vi "Get Array Value at Index - String.vi"(0 "JSON Tree In (JSON Array)":variant, 5 "Index":i32, 9 "Default Value if JSON Null":string, 11 "error in (no error)":errorcluster) -> (4 "JSON Tree Out Passthrough":variant, 6 "String Value":string, 10 "is JSON Null?":bool, 15 "error out":errorcluster)   [LabVIEW 2015, in "i3-json.lvlib"]
doc: "Use this template to build a VI to use as a subVI."
uses:
  i3-json.lvlib
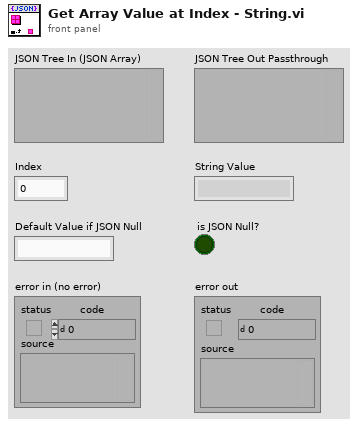
[diagram p1: front panel]
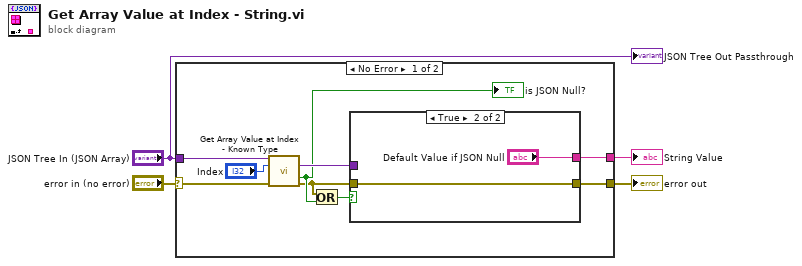
[diagram p0: block diagram]
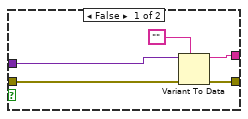
[diagram p2: hidden frame]
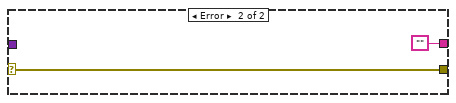
[diagram p3: hidden frame]
diagram:
  n1 = case shown="No Error" "error in (no error)" {
    selector: "error in (no error)" -> [w11 w22]
    tunnel: [w9 w22] -> w3
    tunnel: "JSON Tree In (JSON Array)" -> [w13 _]
    tunnel: [w6 ""] -> w2
    frame No Error {
      n2 = call "Get Array Value at Index - Known Type.vi"("JSON Tree In (JSON Array)"=w13, "Index"="Index", "error in (no error)"=w11) -> ("Value"=w8:variant, "is JSON Null?"=w7:bool, "error out"=w5:errorcluster)  [unwired: 7 in, 3 out]
      "is JSON Null?" <- w7
      n3 = Or(x=w5, y=w7) -> (x .or. y?=w10:bool)
      n4 = case shown="True" w10 {
        tunnel: w5 -> [w18 w20]
        tunnel: [w15 w20] -> w9
        tunnel: w8 -> [w17 _]
        tunnel: [w16 "Default Value if JSON Null"] -> w6
        frame False {
          n5 = Variant To Data(error in=w18, type="" ("Double Value"), Variant=w17) -> (data=w16:string, error out=w15:errorcluster)
        }
        frame True {
        }
      }
    }
    frame Error {
    }
  }
  "error out" <- w3
  "String Value" <- w2
  "JSON Tree Out Passthrough" <- "JSON Tree In (JSON Array)"
